vi "ARB LOAD WFM1.vi"(4 "READ ONLY (T)":bool, 6 "OPC?)T)":bool, 8 "error in":errorcluster {"code" format="%.0x"}, 9 "Timeout":u32=3000, 10 "WRITE WFM1":string="E-TM1_1__10MHZ.WFM", 11 "Session In":refnum<visa-resource-name>="GPIB0::19::INSTR") -> (0 "error out":errorcluster {"code" format="%.0x"}, 2 "READ WFM1":string, 3 "Session Out":refnum<visa-resource-name>)   [LabVIEW 2018]
uses:
  Agilent PSG MXG Series/Agilent PSG MXG Series.lvlib
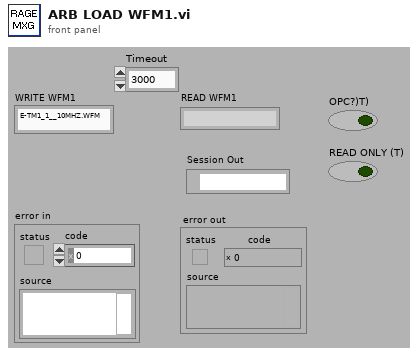
[diagram p1: front panel]
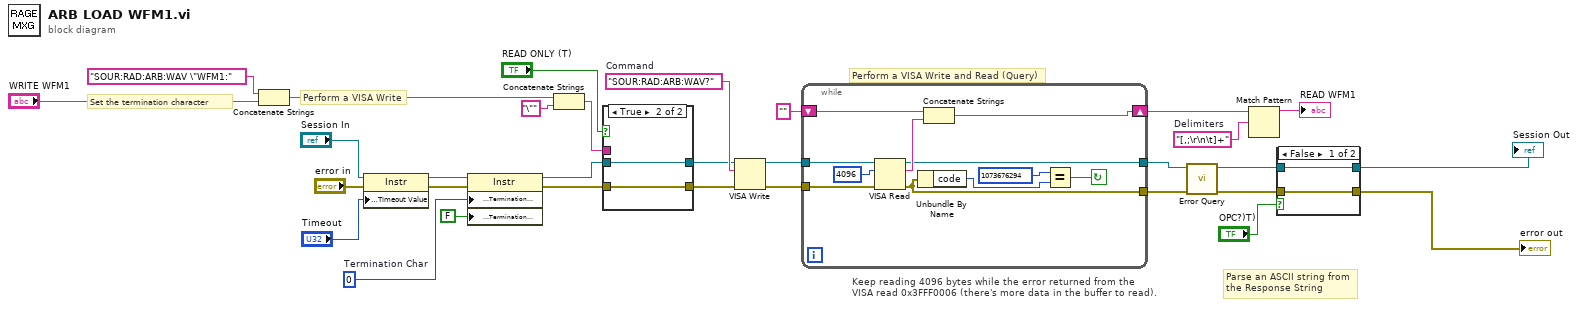
[diagram p0: block diagram]
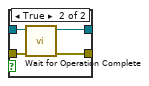
[diagram p2: hidden frame]
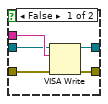
[diagram p3: hidden frame]
diagram:
  w12 = "[,;\r\n\t]+"  # Delimiters
  w14 = "SOUR:RAD:ARB:WAV?"  # Command
  w26 = u8 0  # Termination Char
  # "Parse an ASCII string from the Response String"
  # "Perform a VISA Write and Read (Query)"
  # "Keep reading 4096 bytes while the error returned from the\nVISA read 0x3FFF0006 (there's more data in the buffer to read)."
  # "Perform a VISA Write"
  # "Set the termination character"
  n1 = Concatenate Strings("SOUR:RAD:ARB:WAV \"WFM1:" ("staticText"), "WRITE WFM1") -> (w19:string)
  n2 = property class="Instr"(reference="Session In", error in="error in", "General Settings:Timeout Value"="Timeout") -> (reference out=w25:refnum<visa-resource-name>, error out=w28:errorcluster)
  n3 = property class="Instr"(reference=w25, error in=w28, "Message Based Settings:Termination Character"=w26, "Message Based Settings:Termination Character Enable"=FALSE ("enable")) -> (reference out=w10:refnum<visa-resource-name>, error out=w27:errorcluster)
  n4 = Concatenate Strings(w19, "\"" ("StaticText")) -> (w20:string)
  n5 = case shown="True" "READ ONLY (T)" {
    tunnel: w27 -> [w36 w37]
    tunnel: [w35 w37] -> w21
    tunnel: w20 -> [w34 _]
    tunnel: w10 -> [w33 w38]
    tunnel: [w32 w38] -> w9
    frame False {
      n6 = VISA Write(VISA resource name=w33, write buffer=w34, error in (no error)=w36) -> (VISA resource name out=w32:refnum<visa-resource-name>, error out=w35:errorcluster)  [unwired: 1 out]
    }
    frame True {
    }
  }
  n7 = VISA Write(VISA resource name=w9, write buffer=w14, error in (no error)=w21) -> (VISA resource name out=w17:refnum<visa-resource-name>, error out=w16:errorcluster)  [unwired: 1 out]
  n8 = while {
    tunnel: w17 -> [w46]
    shift-right: [w40] -> w11
    shift-left: "" -> [w45]
    tunnel: w16 -> [w43]
    tunnel: [w42] -> w6
    tunnel: [w39] -> w5
    stop <- w41 continue-if-true
    n9 = VISA Read(VISA resource name=w46, byte count=u32 4096 ("byte count (0)"), error in (no error)=w43) -> (VISA resource name out=w39:refnum<visa-resource-name>, read buffer=w44:string, error out=w42:errorcluster)  [unwired: 1 out]
    n10 = Unbundle By Name(w42) -> ("code"=w48:i32)
    n11 = Concatenate Strings(w45, w44) -> (w40:string)
    n12 = Equal?(x=1073676294, y=w48) -> (x = y?=w41:bool)
  }
  n13 = call "Error Query.vi"("error in (no error)"=w6, "VISA resource name"=w5) -> ("error out"=w7:errorcluster, "VISA resource name out"=w2:refnum<visa-resource-name>)  [unwired: 6 in, 2 out]
  n14 = Match Pattern(string=w11, regular expression=w12) -> (before substring=→"READ WFM1":string)  [unwired: 4 out]
  n15 = case shown="False" "OPC?)T)" {
    tunnel: w7 -> [w51 w55]
    tunnel: [w51 w54] -> w4
    tunnel: [w50 w53] -> w3
    tunnel: w2 -> [w50 w52]
    frame False {
    }
    frame True {
      n16 = call "Wait for Operation Complete.vi"("error in (no error)"=w55, "VISA resource name"=w52) -> ("error out"=w54:errorcluster, "VISA resource name out"=w53:refnum<visa-resource-name>)  [unwired: 8 in]
    }
  }
  "error out" <- w4
  "Session Out" <- w3
